vi "DMSV.subscribe_node_services.vi"(0 "nodeServices":i32[][](array[numeric]), 1 "nodeNotifiers":refnum<notifier>[][](array[refnum]), 2 "nodes":string[](array[string]), 5 "error in (no error)":errorcluster) -> (14 "nodeServices (out)":i32[][](array[numeric]), 15 "nodeNotifiers (out)":refnum<notifier>[][](array[refnum]), 19 "error out":errorcluster)   [LabVIEW 2014, in "DMSViewer.lvlib"]
doc: "Subscribes the domain viewer to DIM services providing information about nodes.\n\nauthor: Dietrich Beck, GSI\n\nLicense Agreement for this software:\n\nCopyright (C)\nGesellschaft für Schwerionenforschung, GSI\nPlanckstr. 1\n64291 Darmstadt\nGermany\n\nContact: D.Beck@gsi.de \n\nThis program is free software; you can redistribute it and/or modify it under the terms of the GNU General Public License as published by the Free Software Foundation; either version 2 of the license, or (at your option) any later version.\n\nThis program is distributed in the hope that it will be useful, but WITHOUT ANY WARRANTY; without even the implied warranty of MERCHANTABILITY or FITNESS FOR A PARTICULAR PURPOSE. See the GNU General License for more details (http://www.gnu.org).\n\nGesellschaft für Schwerionenforschung, GSI\nPlanckstr. 1, 64291 Darmstadt, Germany\nFor all questions and ideas contact: M.Richter@gsi.de, H.Brand@gsi.de or D.Beck@gsi.de.\nLast update: 10-OCT-2004"
uses:
  DMSViewer.lvlib
  CSlibraries-extern/DimLVEvent/LVDimInterface/LVDimInterface.dim service type.ctl
  CSlibraries-extern/DimLVEvent/LVDimInterface/LVDimInterface.dic_info_service_notifier.vi
  CSlibraries-extern/DimLVEvent/LVDimInterface/LVDimInterface.lvlib
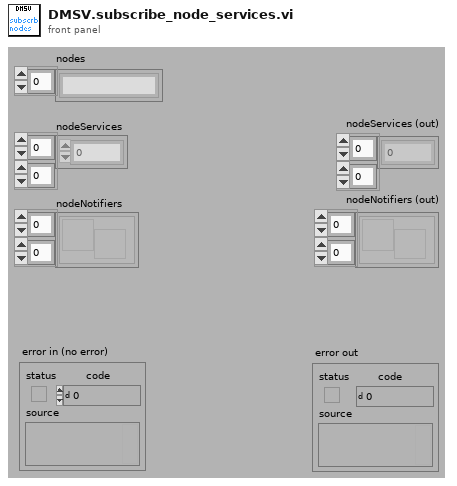
[diagram p1: front panel]
types:
  T1 = typedef "LVDimInterface.lvlib/LVDimInterface.dim service type.ctl" = u16
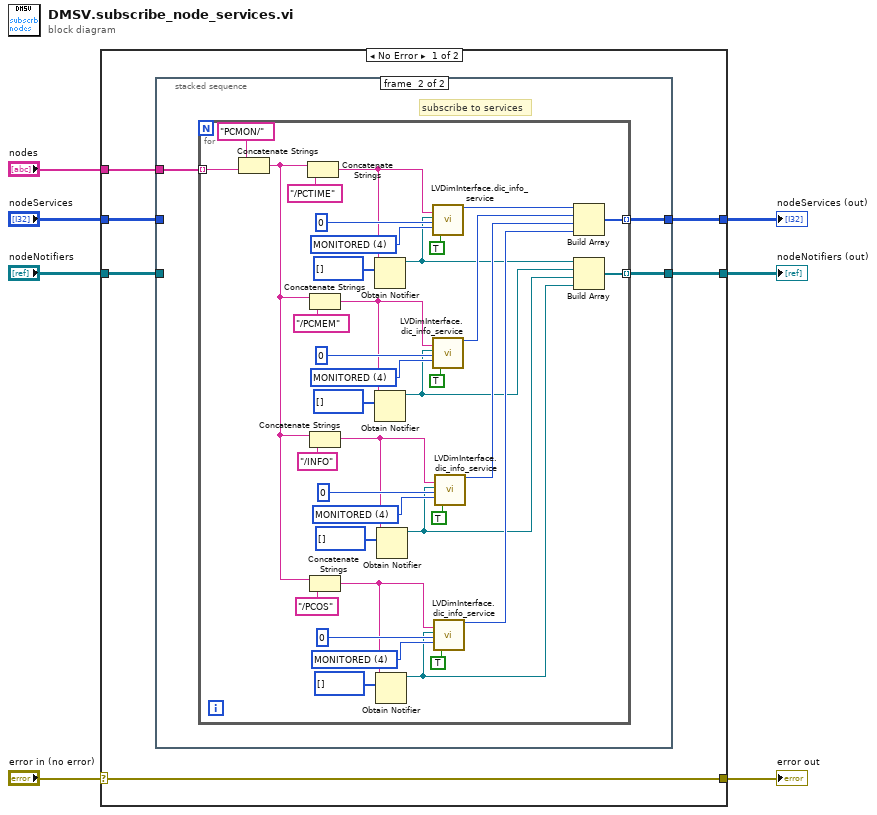
[diagram p0: block diagram]
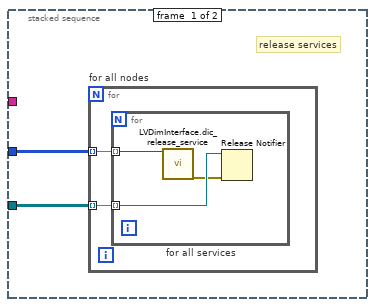
[diagram p2: hidden frame]
diagram:
  n1 = case shown="No Error" "error in (no error)" {
    selector: "error in (no error)" -> [w8 w63]
    tunnel: "nodes" -> [w13 _]
    tunnel: [w8 w63] -> w5
    tunnel: [w12 w62] -> w4
    tunnel: [w11 w61] -> w3
    tunnel: "nodeServices" -> [w10 w62]
    tunnel: "nodeNotifiers" -> [w9 w61]
    frame No Error {
      n2 = stacked-sequence {
        tunnel: w13 -> [_ w23]
        tunnel: [_ w22] -> w12
        tunnel: [_ w21] -> w11
        tunnel: w10 -> [w15 _]
        tunnel: w9 -> [w14 _]
        frame #0 {
          # "release services"
          n3 = for "for all nodes" {
            tunnel: w15 -> [w17] mode=indexing
            tunnel: w14 -> [w16] mode=indexing
            n4 = for "for all services" {
              tunnel: w17 -> [w20] mode=indexing
              tunnel: w16 -> [w19] mode=indexing
              n5 = call "LVDimInterface.dic_release_service.vi"("callBackID"=w20) -> ("error out"=w18:errorcluster)  [unwired: 18 in]
              n6 = Release Notifier(notifier=w19, error in (no error)=w18) -> ()  [unwired: 1 in, 3 out]
            }
          }
        }
        frame #1 {
          # "subscribe to services"
          n7 = for {
            tunnel: w23 -> [w54] mode=indexing
            tunnel: [w25] -> w22 mode=indexing
            tunnel: [w24] -> w21 mode=indexing
            w37 = T1 4 items=["ONCE_ONLY"=1, "TIMED"=2, "MONITORED"=4] ("serviceType")
            w41 = T1 4 items=["ONCE_ONLY"=1, "TIMED"=2, "MONITORED"=4] ("serviceType")
            w47 = T1 4 items=["ONCE_ONLY"=1, "TIMED"=2, "MONITORED"=4] ("serviceType")
            w51 = T1 4 items=["ONCE_ONLY"=1, "TIMED"=2, "MONITORED"=4] ("serviceType")
            n8 = Concatenate Strings("PCMON/" ("string"), w54) -> (w55:string)
            n9 = Concatenate Strings(w55, "/PCTIME" ("string")) -> (w49:string)
            n10 = Concatenate Strings(w55, "/PCMEM" ("string")) -> (w44:string)
            n11 = Concatenate Strings(w55, "/INFO") -> (w39:string)
            n12 = Concatenate Strings(w55, "/PCOS") -> (w34:string)
            n13 = Obtain Notifier(name (unnamed)=w49, notification data type=i8[] []) -> (notifier out=w29:refnum<notifier>)  [unwired: 2 in, 2 out]
            n14 = Obtain Notifier(name (unnamed)=w44, notification data type=i8[] []) -> (notifier out=w28:refnum<notifier>)  [unwired: 2 in, 2 out]
            n15 = Obtain Notifier(name (unnamed)=w34, notification data type=i8[] []) -> (notifier out=w26:refnum<notifier>)  [unwired: 2 in, 2 out]
            n16 = Obtain Notifier(name (unnamed)=w39, notification data type=i8[] []) -> (notifier out=w27:refnum<notifier>)  [unwired: 2 in, 2 out]
            n17 = call-poly "LVDimInterface.dic_info_service.vi"("serviceName"=w49, "notifierRef"=w29, "timeout [s]"=0, "serviceType"=w51, "stamped"=TRUE) -> ("callBackID"=w33:i32)  [unwired: 13 in, 1 out]
            n18 = call-poly "LVDimInterface.dic_info_service.vi"("serviceName"=w44, "notifierRef"=w28, "timeout [s]"=0, "serviceType"=w47, "stamped"=TRUE) -> ("callBackID"=w32:i32)  [unwired: 13 in, 1 out]
            n19 = call-poly "LVDimInterface.dic_info_service.vi"("serviceName"=w34, "notifierRef"=w26, "timeout [s]"=0, "serviceType"=w37, "stamped"=TRUE) -> ("callBackID"=w30:i32)  [unwired: 13 in, 1 out]
            n20 = call-poly "LVDimInterface.dic_info_service.vi"("serviceName"=w39, "notifierRef"=w27, "timeout [s]"=0, "serviceType"=w41, "stamped"=TRUE) -> ("callBackID"=w31:i32)  [unwired: 13 in, 1 out]
            n21 = Build Array(w33, w32, w31, w30) -> (w25:i32[])
            n22 = Build Array(w29, w28, w27, w26) -> (w24:refnum<notifier>[])
          }
        }
      }
    }
    frame Error {
    }
  }
  "error out" <- w5
  "nodeServices (out)" <- w4
  "nodeNotifiers (out)" <- w3
